vi "LABVIWE_FLAT_SQEQUENCE.vi"() -> ()   [LabVIEW 2020]
panel:
  out "Numeric 3":dbl
  in  "Numeric 2":dbl
  in  "Numeric":dbl
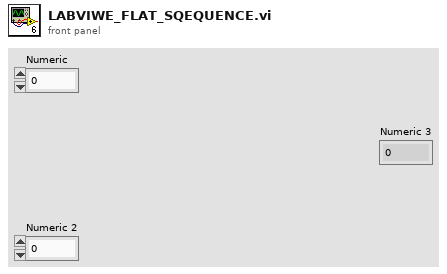
[diagram p1: front panel]
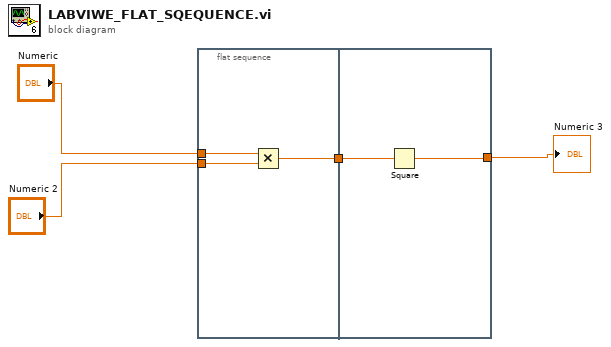
[diagram p0: block diagram]
diagram:
  n1 = flat-sequence {
    tunnel: "Numeric" -> [w7]
    tunnel: "Numeric 2" -> [w6]
    tunnel: [w5] -> w2
    tunnel: w2 -> [w9]
    tunnel: [w8] -> w1
    frame #0 {
      n2 = Multiply(x=w7, y=w6) -> (x*y=w5:dbl)
    }
    frame #1 {
      n3 = Square(x=w9) -> (x^2=w8:dbl)
    }
  }
  "Numeric 3" <- w1
